vi "1.Bounce Window_System Configuration.vi"(11 "群組：":T1) -> (3 "系統管理選單":T2)   [LabVIEW 2015]
uses:
  0.Main_Control/Control_Bounce Window_Main_System Configuration.ctl
  <vilib>/Utility/miscctls.llb/LVPointTypeDef.ctl
panel:
  in  "離開":bool
  in  "機器參數設定":bool
  in  "手動操作":bool
  in  "帳號管理":bool
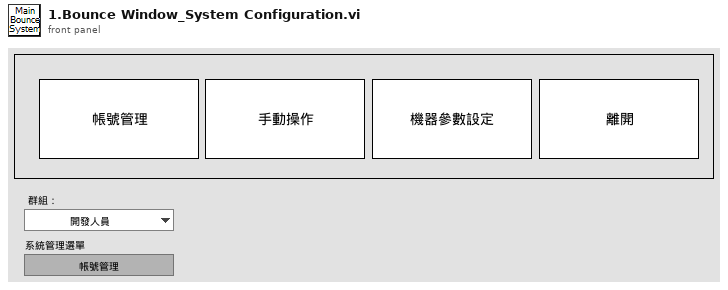
[diagram p1: front panel]
types:
  T1 = typedef "Control_User account_Permissions.ctl" = enum16{"開發人員", "管理者", "工程師", "作業員"}
  T2 = typedef "Control_Bounce Window_Main_System Configuration.ctl" = enum16{"帳號管理", "手動操作", "機器參數設定", "離開", "等待"}
  T3 = typedef "LVPointTypeDef.ctl" = cluster{"Horizontal":i16, "Vertical":i16}
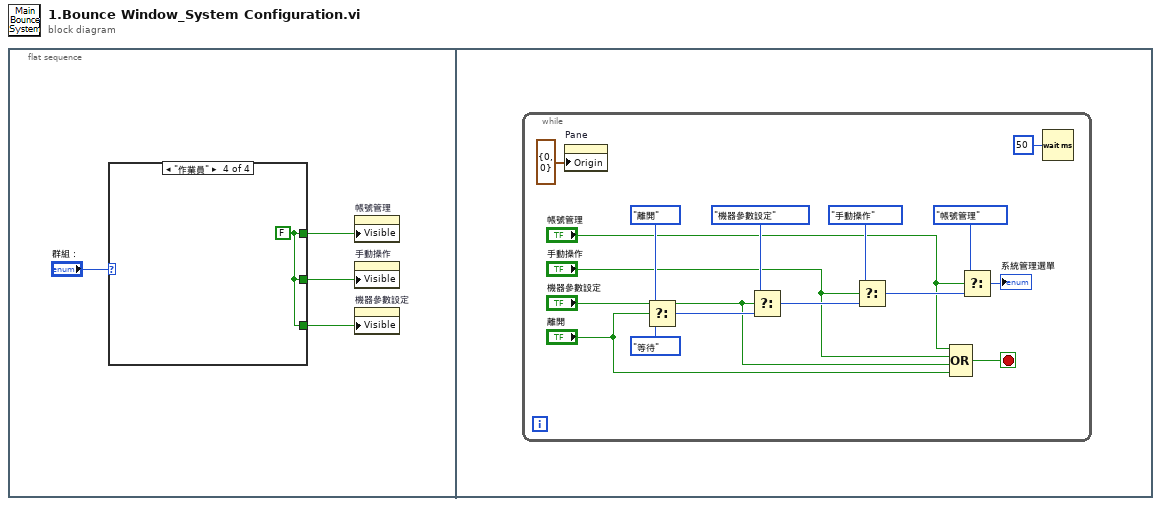
[diagram p0: block diagram]
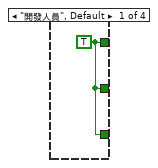
[diagram p2: hidden frame]
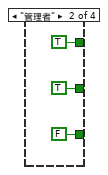
[diagram p3: hidden frame]
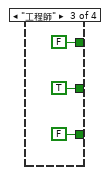
[diagram p4: hidden frame]
diagram:
  n1 = flat-sequence {
    frame #0 {
      n2 = case shown="\"作業員\"" "群組：" {
        tunnel: [w5 FALSE FALSE w12] -> w3
        tunnel: [w5 TRUE FALSE w12] -> w2
        tunnel: [w5 TRUE TRUE w12] -> w1
        frame "開發人員", Default {
          w5 = TRUE
        }
        frame "管理者" {
        }
        frame "工程師" {
        }
        frame "作業員" {
          w12 = FALSE
        }
      }
      n3 = property on="帳號管理" class="Bool"("Visible"=w2) -> ()  [unwired: 2 in, 2 out]
      n4 = property on="手動操作" class="Bool"("Visible"=w1) -> ()  [unwired: 2 in, 2 out]
      n5 = property on="機器參數設定" class="Bool"("Visible"=w3) -> ()  [unwired: 2 in, 2 out]
    }
    frame #1 {
      n6 = while {
        stop <- w15 stop-if-true
        n7 = property on="Pane" class="Pane"("Origin"=T3 {"Horizontal"=0, "Vertical"=0}) -> ()  [unwired: 2 in, 2 out]
        n8 = Select(t=Control_Bounce_Window_Main_System_Configuration."離開" ("系統管理選單"), s="離開", f=Control_Bounce_Window_Main_System_Configuration."等待" ("系統管理選單")) -> (s? t:f=w25:T2)
        n9 = Select(t=Control_Bounce_Window_Main_System_Configuration."機器參數設定" ("系統管理選單"), s="機器參數設定", f=w25) -> (s? t:f=w23:T2)
        n10 = Select(t=Control_Bounce_Window_Main_System_Configuration."手動操作" ("系統管理選單"), s="手動操作", f=w23) -> (s? t:f=w20:T2)
        n11 = Compound Arithmetic op=OR("帳號管理", "手動操作", "機器參數設定", "離開") -> (w15:bool)
        n12 = Select(t=Control_Bounce_Window_Main_System_Configuration."帳號管理" ("系統管理選單"), s="帳號管理", f=w20) -> (s? t:f=→"系統管理選單":T2)
        n13 = Wait (ms)(milliseconds to wait=u32 50) -> ()  [unwired: 1 out]
      }
    }
  }
